vi "Function 1.vi"(8 "error in (no error)":errorcluster, 10 "Differential_Top":dbl=10.0 format="%#_13g", 11 "Data Cluster":T1={"Vesta Data Output"={"Temp_W_Raw_U"=0, "Temp_W_Raw_L"=0, "Temperature Water (F)"=0.0, "Temperature Water Compensated (F)"=0.0, "Temperature Ambient (F)"=0.0, "Setpoint Location (F)"=0.0, "Heat Request"="", "Fault Ram"="", "PWM DCDC Value"=0, "Pilot Voltage (mV)"=0.0, "Setpoint Actual (F)"=0.0, "Differential Actual (F)"=0.0, "Setpoint User (F)"=0.0, "Differential User (F)"=0.0, "Termperature FIltered -TCO (F)"=0.0, "Temp_C_Raw_1 - Sensor Voltage"="", "Temp_C_Raw_2 - Sensor Voltage"="", "Chamber Sensor Temperature (F)"=0.0, "LDO Base Temperature (F)"=0.0, "LDO Timer (sec)"=0, "Disabled (0)"=FALSE, "Warming (1)"=FALSE, "Heating (2)"=FALSE, "Cooling Data Write (3)"=FALSE, "Cooling (4)"=FALSE, "Data Read (5)"=FALSE, "N/A"=FALSE, "Temperature Trip (7)"=FALSE, "Burner"=FALSE}, "VestaTemperature"={"Water Heater Temp (°F)"=135, "Differential  (°F)"=10.0}, "Timer Application Data"={"Duty Cycle"={"Burner ON Time (Seconds)"=60.0, "Burner OFF Time (Seconds)"=60.0, "Main Burner Flag"=FALSE, "Burner Power Mode"=0}}, "Data Array"=[], "MW Output"={"TC1-Channel 021"=0.0, "TC2-Channel 022"=0.0, "TC3-Channel 023"=0.0, "TC4-Channel 024"=0.0, "TC5-Channel 025"=0.0, "TC6-Channel 026"=0.0, "TC7-Channel 017"=0.0, "TC8-Channel 028"=0.0, "TC9-Channel 029"=0.0, "TC10-Channel 030"=0.0, "TC Tree Average"=0.0, "TC DWN- Channel 027"=0.0, "RTDin-Channel 031"=0.0, "RTDout-Channel 032"=0.0, "RTDamb-Channel 033"=0.0, "PSI1-Channel 011"=0.0, "PSI2-Channel 012"=0.0, "PSI3-Channel 013"=0.0, "PSI4-Channel 014"=0.0, "UE State-Channel 015"=0.0, "LE State-Channel 016"=0.0, "Module 4 Relay Status Output"={"INTELLIFAUCET TEMP(T)/FLOW(F) (CH 041)"=FALSE, "INTELLIFAUCET READY (CH 042)"=FALSE, "INTELLIFAUCET START (CH 043)"=FALSE, "INTELLIFAUCET STOP (CH 044)"=FALSE, "MAIN POWER RELAY (CH 047)"=FALSE, "NOT USED (CH 045)"=FALSE, "NOT USED (CH 046)"=FALSE, "PURGE VALVE RELAY (CH 048)"=FALSE, "OUTLET VALVE RELAY (CH 049)"=FALSE, "INLET VALVE RELAY (CH 050)"=FALSE, "Intellifaucet (% Open)"=0.0, "Proportioning Valve (%Open)"=0.0, "Intellifaucet Temp Setpoint (F)"=0.0}}} {"VestaTemperature"."Water Heater Temp (°F)" min=32 max=203}) -> (0 "error out":errorcluster, 3 "Data Cluster Out":T1={"Vesta Data Output"={"Temp_W_Raw_U"=0, "Temp_W_Raw_L"=0, "Temperature Water (F)"=0.0, "Temperature Water Compensated (F)"=0.0, "Temperature Ambient (F)"=0.0, "Setpoint Location (F)"=0.0, "Heat Request"="", "Fault Ram"="", "PWM DCDC Value"=0, "Pilot Voltage (mV)"=0.0, "Setpoint Actual (F)"=0.0, "Differential Actual (F)"=0.0, "Setpoint User (F)"=0.0, "Differential User (F)"=0.0, "Termperature FIltered -TCO (F)"=0.0, "Temp_C_Raw_1 - Sensor Voltage"="", "Temp_C_Raw_2 - Sensor Voltage"="", "Chamber Sensor Temperature (F)"=0.0, "LDO Base Temperature (F)"=0.0, "LDO Timer (sec)"=0, "Disabled (0)"=FALSE, "Warming (1)"=FALSE, "Heating (2)"=FALSE, "Cooling Data Write (3)"=FALSE, "Cooling (4)"=FALSE, "Data Read (5)"=FALSE, "N/A"=FALSE, "Temperature Trip (7)"=FALSE, "Burner"=FALSE}, "VestaTemperature"={"Water Heater Temp (°F)"=135, "Differential  (°F)"=10.0}, "Timer Application Data"={"Duty Cycle"={"Burner ON Time (Seconds)"=60.0, "Burner OFF Time (Seconds)"=60.0, "Main Burner Flag"=FALSE, "Burner Power Mode"=0}}, "Data Array"=[], "MW Output"={"TC1-Channel 021"=0.0, "TC2-Channel 022"=0.0, "TC3-Channel 023"=0.0, "TC4-Channel 024"=0.0, "TC5-Channel 025"=0.0, "TC6-Channel 026"=0.0, "TC7-Channel 017"=0.0, "TC8-Channel 028"=0.0, "TC9-Channel 029"=0.0, "TC10-Channel 030"=0.0, "TC Tree Average"=0.0, "TC DWN- Channel 027"=0.0, "RTDin-Channel 031"=0.0, "RTDout-Channel 032"=0.0, "RTDamb-Channel 033"=0.0, "PSI1-Channel 011"=0.0, "PSI2-Channel 012"=0.0, "PSI3-Channel 013"=0.0, "PSI4-Channel 014"=0.0, "UE State-Channel 015"=0.0, "LE State-Channel 016"=0.0, "Module 4 Relay Status Output"={"INTELLIFAUCET TEMP(T)/FLOW(F) (CH 041)"=FALSE, "INTELLIFAUCET READY (CH 042)"=FALSE, "INTELLIFAUCET START (CH 043)"=FALSE, "INTELLIFAUCET STOP (CH 044)"=FALSE, "MAIN POWER RELAY (CH 047)"=FALSE, "NOT USED (CH 045)"=FALSE, "NOT USED (CH 046)"=FALSE, "PURGE VALVE RELAY (CH 048)"=FALSE, "OUTLET VALVE RELAY (CH 049)"=FALSE, "INLET VALVE RELAY (CH 050)"=FALSE, "Intellifaucet (% Open)"=0.0, "Proportioning Valve (%Open)"=0.0, "Intellifaucet Temp Setpoint (F)"=0.0}}} {"VestaTemperature"."Water Heater Temp (°F)" min=32 max=203}, 4 "Send_Vesta_Message":u8)   [LabVIEW 2023]
uses:
  controls/UI Data.ctl
  Drivers/Resideo Gas Valve/Type Definitions/Vesta Info.ctl
  Drivers/Resideo Gas Valve/Type Definitions/Temperature Control.ctl
  controls/Timer Application Cluster.ctl
  controls/Burner Duty Cycle.ctl
  Hybrid Water Heater/Type Definitions/HEWH MW100 Data Cluster.ctl
  Hybrid Water Heater/Custom Instrument Control/MW100/Type Definitions/HEWH Module 4 Relay Status.ctl
  <vilib>/Utility/error.llb/whitespace.ctl
  <vilib>/Utility/error.llb/Trim Whitespace One-Sided.vi
panel:
  out "Burner":i16
  out "Power_Mode_Out":u8
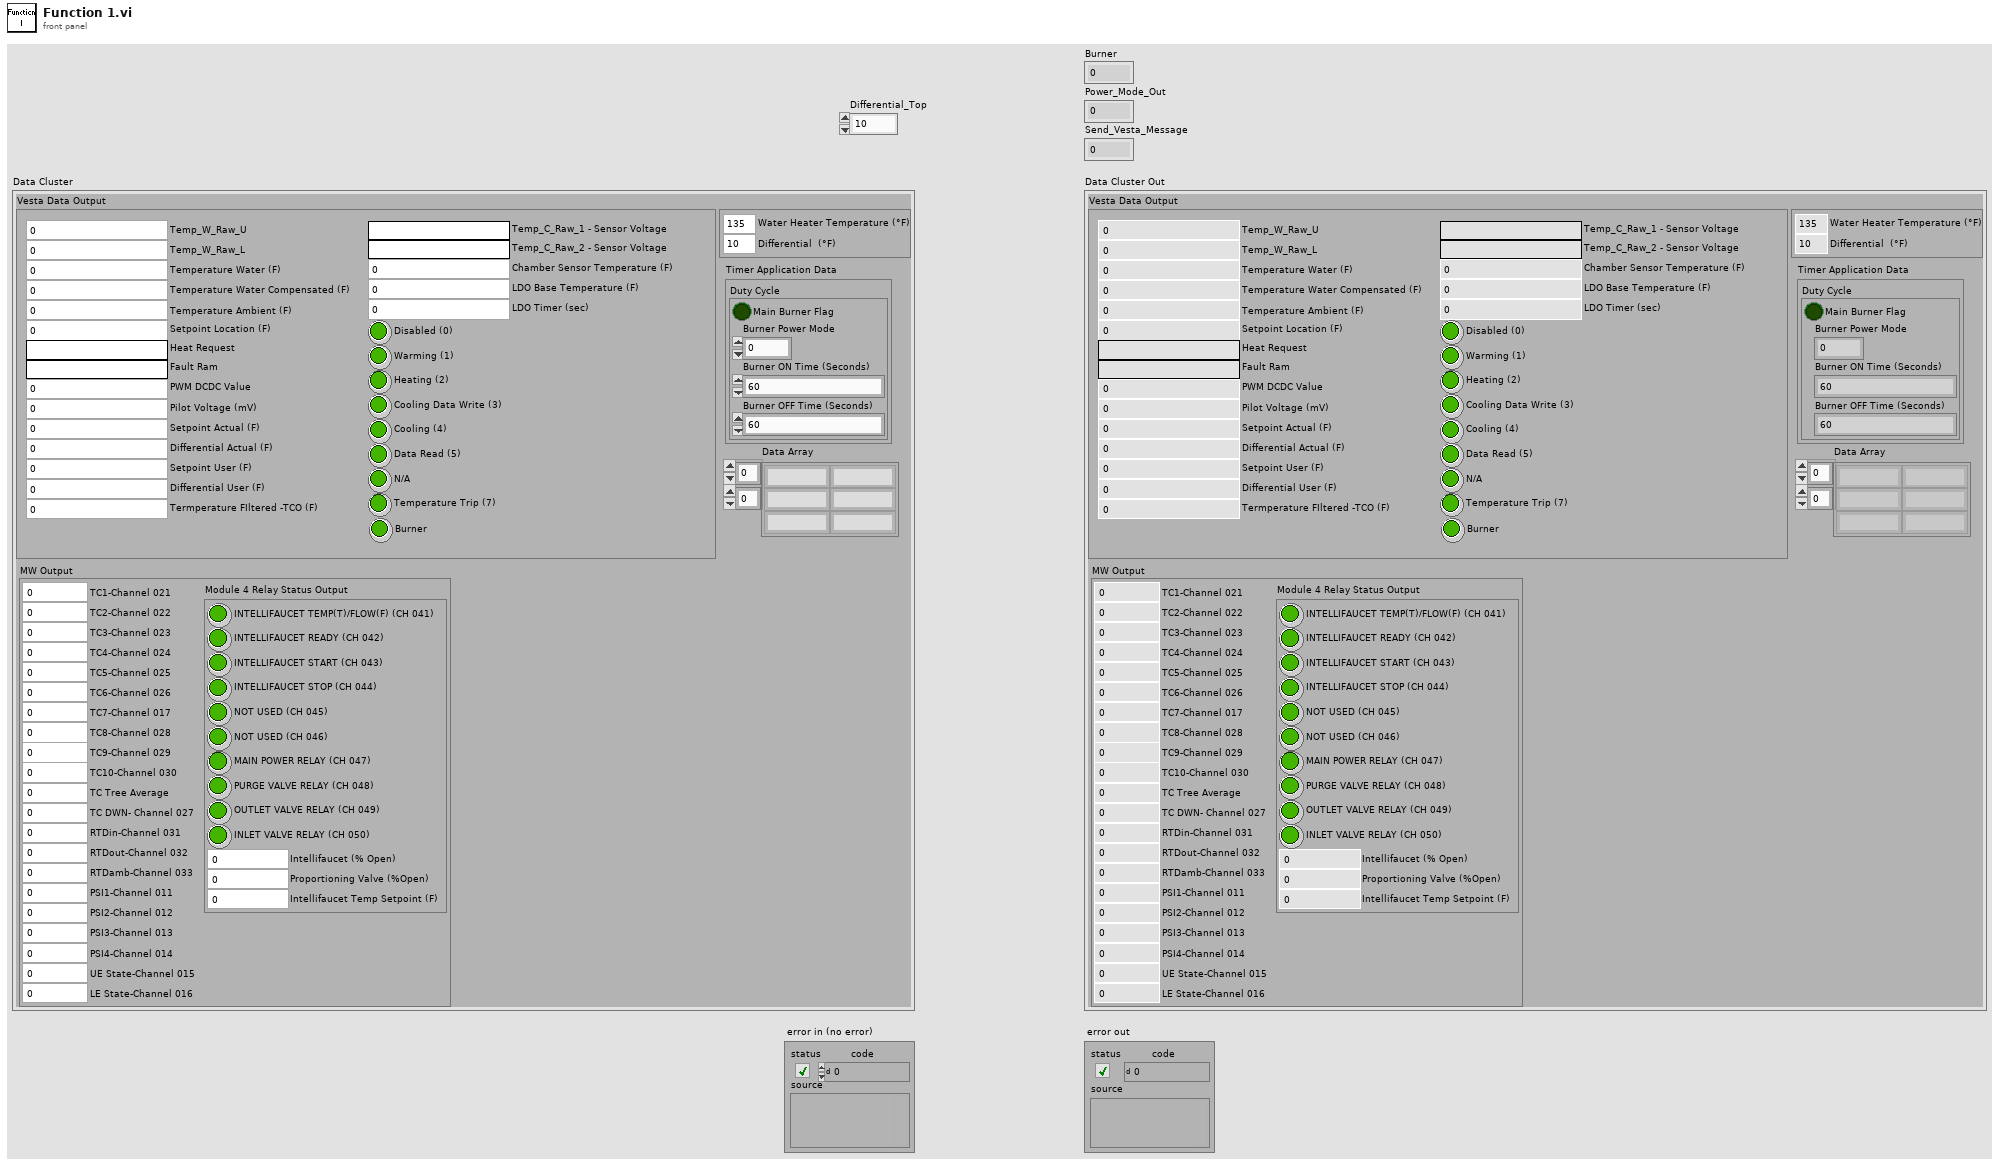
[diagram p1: front panel]
types:
  T1 = typedef "UI Data.ctl" = cluster{"Vesta Data Output":T2, "VestaTemperature":T3, "Timer Application Data":T4, "Data Array":string[][], "MW Output":T6}
  T2 = typedef "Vesta Info.ctl" = cluster{"Temp_W_Raw_U":u16, "Temp_W_Raw_L":u16, "Temperature Water (F)":dbl, "Temperature Water Compensated (F)":dbl, "Temperature Ambient (F)":dbl, "Setpoint Location (F)":dbl, "Heat Request":string, "Fault Ram":string, "PWM DCDC Value":u16, "Pilot Voltage (mV)":dbl, "Setpoint Actual (F)":dbl, "Differential Actual (F)":dbl, "Setpoint User (F)":dbl, "Differential User (F)":dbl, "Termperature FIltered -TCO (F)":dbl, "Temp_C_Raw_1 - Sensor Voltage":string, "Temp_C_Raw_2 - Sensor Voltage":string, "Chamber Sensor Temperature (F)":dbl, "LDO Base Temperature (F)":dbl, "LDO Timer (sec)":i16, "Disabled (0)":bool, "Warming (1)":bool, "Heating (2)":bool, "Cooling Data Write (3)":bool, "Cooling (4)":bool, "Data Read (5)":bool, "N/A":bool, "Temperature Trip (7)":bool, "Burner":bool}
  T3 = typedef "Temperature Control.ctl" = cluster{"Water Heater Temp (°F)":u16, "Differential  (°F)":dbl}
  T4 = typedef "Timer Application Cluster.ctl" = cluster{"Duty Cycle":T5}
  T5 = typedef "Burner Duty Cycle.ctl" = cluster{"Burner ON Time (Seconds)":dbl, "Burner OFF Time (Seconds)":dbl, "Main Burner Flag":bool, "Burner Power Mode":u8}
  T6 = typedef "HEWH MW100 Data Cluster.ctl" = cluster{"TC1-Channel 021":dbl, "TC2-Channel 022":dbl, "TC3-Channel 023":dbl, "TC4-Channel 024":dbl, "TC5-Channel 025":dbl, "TC6-Channel 026":dbl, "TC7-Channel 017":dbl, "TC8-Channel 028":dbl, "TC9-Channel 029":dbl, "TC10-Channel 030":dbl, "TC Tree Average":dbl, "TC DWN- Channel 027":dbl, "RTDin-Channel 031":dbl, "RTDout-Channel 032":dbl, "RTDamb-Channel 033":dbl, "PSI1-Channel 011":dbl, "PSI2-Channel 012":dbl, "PSI3-Channel 013":dbl, "PSI4-Channel 014":dbl, "UE State-Channel 015":dbl, "LE State-Channel 016":dbl, "Module 4 Relay Status Output":T7}
  T7 = typedef "HEWH Module 4 Relay Status.ctl" = cluster{"INTELLIFAUCET TEMP(T)/FLOW(F) (CH 041)":bool, "INTELLIFAUCET READY (CH 042)":bool, "INTELLIFAUCET START (CH 043)":bool, "INTELLIFAUCET STOP (CH 044)":bool, "MAIN POWER RELAY (CH 047)":bool, "NOT USED (CH 045)":bool, "NOT USED (CH 046)":bool, "PURGE VALVE RELAY (CH 048)":bool, "OUTLET VALVE RELAY (CH 049)":bool, "INLET VALVE RELAY (CH 050)":bool, "Intellifaucet (% Open)":dbl, "Proportioning Valve (%Open)":dbl, "Intellifaucet Temp Setpoint (F)":dbl}
  T8 = typedef "whitespace.ctl" = u16
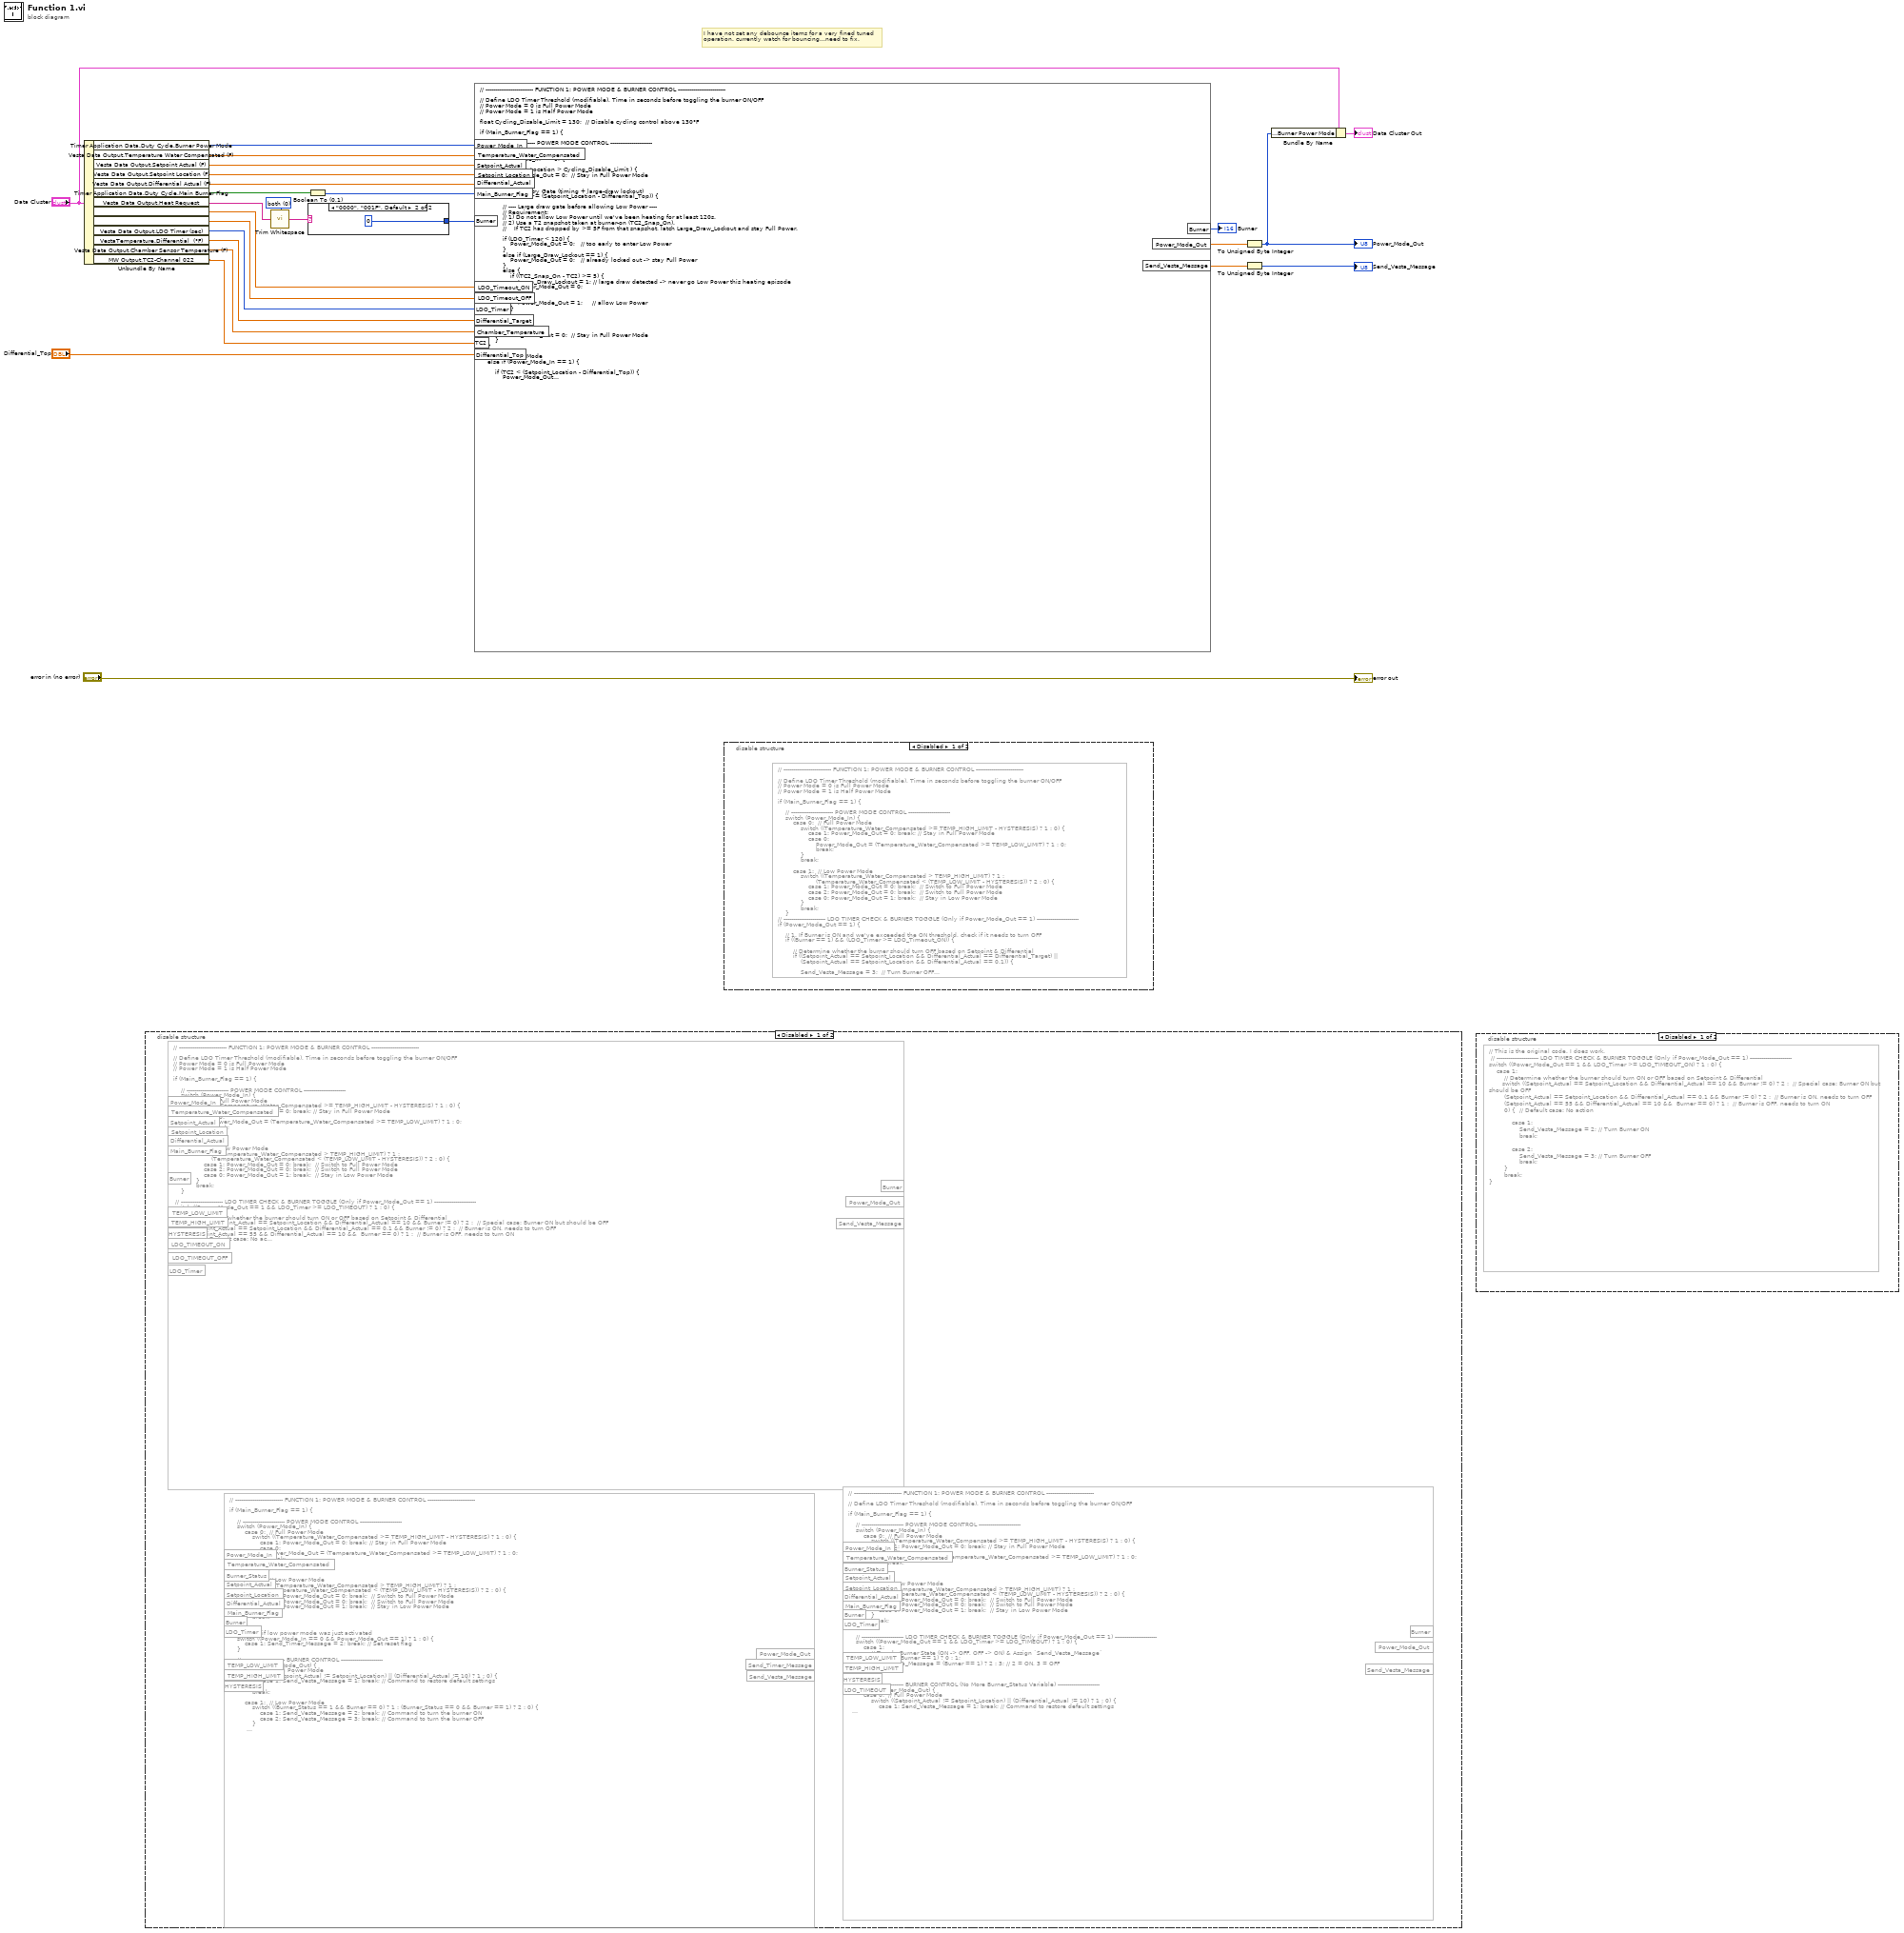
[diagram p0: block diagram]
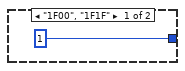
[diagram p4: hidden frame]
diagram:
  w9 = T8 0 items=["both", "start of string", "end of string"] ("location (both)")
  # "I have not set any debounce items for a very fined tuned \noperation. currently watch for bouncing...need to fix."
  n1 = Unbundle By Name("Data Cluster") -> ("Timer Application Data.Duty Cycle.Burner Power Mode"=w20:u8, "Vesta Data Output.Temperature Water Compensated (F)"=w19:dbl, "Vesta Data Output.Setpoint Actual (F)"=w24:dbl, "Vesta Data Output.Setpoint Location (F)"=w23:dbl, "Vesta Data Output.Differential Actual (F)"=w22:dbl, "Timer Application Data.Duty Cycle.Main Burner Flag"=w26:bool, "Vesta Data Output.Heat Request"=w10:string, "Timer Application Data.Duty Cycle.Burner ON Time (Seconds)"=w7:dbl, "Timer Application Data.Duty Cycle.Burner OFF Time (Seconds)"=w6:dbl, "Vesta Data Output.LDO Timer (sec)"=w12:i16, "VestaTemperature.Differential  (°F)"=w4:dbl, "Vesta Data Output.Chamber Sensor Temperature (F)"=w3:dbl, "MW Output.TC2-Channel 022"=w2:dbl)
  n2 = disable-structure shown="Disabled" {
    frame Disabled {
      n3 = formula code="// ------------------------- FUNCTION 1: POWER MODE & BURNER CONTROL -------------------------\n\n// Define LDO Timer Threshold (modifiable), Time in seconds before toggling the burner ON/OFF\n// Power Mode = 0 is Full Power Mode\n// Power Mode = 1 is Half Power Mode\n\nif (Main_Burner_Flag == 1) {\n\n    // ---------------------- POWER MODE CONTROL ----------------------\n    switch (Power_Mode_In) {\n        case 0:  // Full Power Mode\n            switch ((Temperature_Water_Compensated >= TEMP_HIGH_LIMIT - HYSTERESIS) ? 1 : 0) {\n                case 1: Power_Mode_Out = 0; break; // Stay in Full Power Mode\n                case 0:\n                    Power_Mode_Out = (Temperature_Water_Compensated >= TEMP_LOW_LIMIT) ? 1 : 0;\n                    break;\n            }\n            break;\n\n        case 1:  // Low Power Mode\n            switch ((Temperature_Water_Compensated > TEMP_HIGH_LIMIT) ? 1 : \n                    (Temperature_Water_Compensated < (TEMP_LOW_LIMIT - HYSTERESIS)) ? 2 : 0) {\n                case 1: Power_Mode_Out = 0; break;  // Switch to Full Power Mode\n                case 2: Power_Mode_Out = 0; break;  // Switch to Full Power Mode\n                case 0: Power_Mode_Out = 1; break;  // Stay in Low Power Mode\n            }\n            break;\n    }\n\n // ---------------------- LDO TIMER CHECK & BURNER TOGGLE (Only if Power_Mode_Out == 1) ----------------------\nswitch ((Power_Mode_Out == 1 && LDO_Timer >= LDO_TIMEOUT) ? 1 : 0) {\n    case 1:\n        // Determine whether the burner should turn ON or OFF based on Setpoint & Differential\n       switch ((Setpoint_Actual == Setpoint_Location && Differential_Actual == 10 && Burner != 0) ? 2 :  // Special case: Burner ON but should be OFF\n        (Setpoint_Actual == Setpoint_Location && Differential_Actual == 0.1 && Burner != 0) ? 2 :  // Burner is ON, needs to turn OFF\n        (Setpoint_Actual == 55 && Differential_Actual == 10 &&  Burner == 0) ? 1 :  // Burner is OFF, needs to turn ON\n        0) {  // Default case: No action\n\n            case 1:  \n                Send_Vesta_Message = 2; // Turn Burner ON\n                break;\n\n            case 2:\n                Send_Vesta_Message = 3; // Turn Burner OFF\n                break;\n        }\n        break;\n}\n\n    // ---------------------- BURNER CONTROL (No More Burner_Status Variable) ----------------------\n    switch (Power_Mode_Out) {\n        case 0:  // Full Power Mode\n            switch ((Setpoint_Actual != Setpoint_Location) || (Differential_Actual != 10) ? 1 : 0) {\n                case 1: Send_Vesta_Message = 1; break; // Command to restore default settings\n            }\n            break;\n    }\n}"() -> ()  [unwired: 13 in, 3 out]
      n4 = formula code="// ------------------------- FUNCTION 1: POWER MODE & BURNER CONTROL -------------------------\n\nif (Main_Burner_Flag == 1) {\n\n    // ---------------------- POWER MODE CONTROL ----------------------\n    switch (Power_Mode_In) {\n        case 0:  // Full Power Mode\n            switch ((Temperature_Water_Compensated >= TEMP_HIGH_LIMIT - HYSTERESIS) ? 1 : 0) {\n                case 1: Power_Mode_Out = 0; break; // Stay in Full Power Mode\n                case 0:\n                    Power_Mode_Out = (Temperature_Water_Compensated >= TEMP_LOW_LIMIT) ? 1 : 0;\n                    break;\n            }\n            break;\n\n        case 1:  // Low Power Mode\n            switch ((Temperature_Water_Compensated > TEMP_HIGH_LIMIT) ? 1 : \n                    (Temperature_Water_Compensated < (TEMP_LOW_LIMIT - HYSTERESIS)) ? 2 : 0) {\n                case 1: Power_Mode_Out = 0; break;  // Switch to Full Power Mode\n                case 2: Power_Mode_Out = 0; break;  // Switch to Full Power Mode\n                case 0: Power_Mode_Out = 1; break;  // Stay in Low Power Mode\n            }\n            break;\n    }\n\n    // Check if low power mode was just activated\n    switch ((Power_Mode_In == 0 && Power_Mode_Out == 1) ? 1 : 0) {\n        case 1: Send_Timer_Message = 2; break; // Set reset flag\n    }\n\n    // ---------------------- BURNER CONTROL ----------------------\n    switch (Power_Mode_Out) {\n        case 0:  // Full Power Mode\n            switch ((Setpoint_Actual != Setpoint_Location) || (Differential_Actual != 10) ? 1 : 0) {\n                case 1: Send_Vesta_Message = 1; break; // Command to restore default settings\n            }\n            break;\n\n        case 1:  // Low Power Mode\n            switch ((Burner_Status == 1 && Burner == 0) ? 1 : (Burner_Status == 0 && Burner == 1) ? 2 : 0) {\n                case 1: Send_Vesta_Message = 2; break; // Command to turn the burner ON\n                case 2: Send_Vesta_Message = 3; break; // Command to turn the burner OFF\n            }\n            break;\n    }\n}"() -> ()  [unwired: 12 in, 3 out]
      n5 = formula code="// ------------------------- FUNCTION 1: POWER MODE & BURNER CONTROL -------------------------\n\n// Define LDO Timer Threshold (modifiable), Time in seconds before toggling the burner ON/OFF\n\nif (Main_Burner_Flag == 1) {\n\n    // ---------------------- POWER MODE CONTROL ----------------------\n    switch (Power_Mode_In) {\n        case 0:  // Full Power Mode\n            switch ((Temperature_Water_Compensated >= TEMP_HIGH_LIMIT - HYSTERESIS) ? 1 : 0) {\n                case 1: Power_Mode_Out = 0; break; // Stay in Full Power Mode\n                case 0:\n                    Power_Mode_Out = (Temperature_Water_Compensated >= TEMP_LOW_LIMIT) ? 1 : 0;\n                    break;\n            }\n            break;\n\n        case 1:  // Low Power Mode\n            switch ((Temperature_Water_Compensated > TEMP_HIGH_LIMIT) ? 1 : \n                    (Temperature_Water_Compensated < (TEMP_LOW_LIMIT - HYSTERESIS)) ? 2 : 0) {\n                case 1: Power_Mode_Out = 0; break;  // Switch to Full Power Mode\n                case 2: Power_Mode_Out = 0; break;  // Switch to Full Power Mode\n                case 0: Power_Mode_Out = 1; break;  // Stay in Low Power Mode\n            }\n            break;\n    }\n\n    // ---------------------- LDO TIMER CHECK & BURNER TOGGLE (Only if Power_Mode_Out == 1) ----------------------\n    switch ((Power_Mode_Out == 1 && LDO_Timer >= LDO_TIMEOUT) ? 1 : 0) {\n        case 1:\n            // Toggle Burner State (ON -> OFF, OFF -> ON) & Assign `Send_Vesta_Message`\n            Burner = (Burner == 1) ? 0 : 1;\n            Send_Vesta_Message = (Burner == 1) ? 2 : 3; // 2 = ON, 3 = OFF\n            break;\n    }\n\n    // ---------------------- BURNER CONTROL (No More Burner_Status Variable) ----------------------\n    switch (Power_Mode_Out) {\n        case 0:  // Full Power Mode\n            switch ((Setpoint_Actual != Setpoint_Location) || (Differential_Actual != 10) ? 1 : 0) {\n                case 1: Send_Vesta_Message = 1; break; // Command to restore default settings\n            }\n            break;\n    }\n}"() -> ()  [unwired: 13 in, 3 out]
    }
    frame Enabled {
    }
  }
  n6 = call <vilib>:"Trim Whitespace.vi"("string"=w10, "location (both)"=w9) -> ("trimmed string"=w8:string)
  n7 = case shown="\"0000\", \"001F\", Default" w8 {
    tunnel: [1 0] -> w11
    frame "1F00", "1F1F" {
    }
    frame "0000", "001F", Default {
    }
  }
  n8 = Boolean To (0,1)(Boolean=w26) -> (0, 1=w21:i16)
  n9 = formula code="// ------------------------- FUNCTION 1: POWER MODE & BURNER CONTROL -------------------------\n\n// Define LDO Timer Threshold (modifiable), Time in seconds before toggling the burner ON/OFF\n// Power Mode = 0 is Full Power Mode\n// Power Mode = 1 is Half Power Mode\n\nfloat Cycling_Disable_Limit = 130;  // Disable cycling control above 130°F\n\nif (Main_Burner_Flag == 1) {\n\n    // ---------------------- POWER MODE CONTROL ----------------------\n    \n   // Full Power Mode\n    if (Power_Mode_In == 0) {  \n        \n        if (Setpoint_Location > Cycling_Disable_Limit ) {\n            Power_Mode_Out = 0;  // Stay in Full Power Mode\n        }  \n\n   // Low Power Entry Gate (timing + large-draw lockout)\n        else if (TC2 >= (Setpoint_Location - Differential_Top)) {\n\n            // ---- Large draw gate before allowing Low Power ----\n            // Requirement:\n            // 1) Do not allow Low Power until we've been heating for at least 120s.\n            // 2) Use a T2 snapshot taken at burner-on (TC2_Snap_On).\n            //    If TC2 has dropped by >= 5F from that snapshot, latch Large_Draw_Lockout and stay Full Power.\n\n            if (LDO_Timer < 120) {\n                Power_Mode_Out = 0;   // too early to enter Low Power\n            }\n            else if (Large_Draw_Lockout == 1) {\n                Power_Mode_Out = 0;   // already locked out -> stay Full Power\n            }\n            else {\n                if ((TC2_Snap_On - TC2) >= 5) {\n                    Large_Draw_Lockout = 1; // large draw detected -> never go Low Power this heating episode\n                    Power_Mode_Out = 0;\n                } \n                else {\n                    Power_Mode_Out = 1;     // allow Low Power\n                }\n            }\n        }\n       \n        else {\n            Power_Mode_Out = 0;  // Stay in Full Power Mode\n        }\n    } \n\n    // Low Power Mode\n    else if (Power_Mode_In == 1) { \n \n        if (TC2 < (Setpoint_Location - Differential_Top)) {\n            Power_Mode_Out = 0;  // Too cold at top -> go back to Full Power (recovery)\n        } \n        else if (TC2 >= Setpoint_Location) {\n            Power_Mode_Out = 0;  // Setpoint reached, exit Low Power Mode\n        }\n        else {\n            Power_Mode_Out = 1;  // Stay in Low Power Mode\n        }\n    }\n}\nelse {Power_Mode_Out = 0;}   // If Main_Burner_Flag ==0, then Power_Mode_Out ==0;\n\n// ---------------------- LDO TIMER CHECK & BURNER TOGGLE (Only if Power_Mode_Out == 1) ----------------------\n// Burner duty cycling corresponds to a generalized combustion-chamber temperature.\n// Right now it’s controlled by a basic timer, but it can be tuned to target a specific temperature.\n// Potentially this could use a table lookup to maximize thermal heat transfer.\n\nif (Power_Mode_Out == 1) {\n\n    // 1. If Burner is ON and we've exceeded the ON threshold, check if it needs to turn OFF\n    if ((Burner == 1) && (LDO_Timer >= LDO_Timeout_ON)) {\n\n        // Determine whether the burner should turn OFF based on Setpoint & Differential\n        if ((Setpoint_Actual == Setpoint_Location && Differential_Actual == Differential_Target) ||\n            (Setpoint_Actual == Setpoint_Location && Differential_Actual == 0.1)) {\n\n            Send_Vesta_Message = 3;  // Turn Burner OFF\n        }\n    }\n\n    // 2. Else if Burner is OFF and we've exceeded the OFF threshold, check if it needs to turn ON\n    else if ((Burner == 0) && (LDO_Timer >= LDO_Timeout_OFF)) {\n\n        // Determine whether the burner should turn ON based on Setpoint & Differential\n        if ((Setpoint_Actual == 55) && (Differential_Actual == Differential_Target)) {\n\n            Send_Vesta_Message = 2;  // Turn Burner ON\n        }\n    }\n}\n\n// ---------------------- BURNER CONTROL (No More Burner_Status Variable) ----------------------\nif (Power_Mode_Out == 0) {  // Full Power Mode\n    \n    if ((Setpoint_Actual != Setpoint_Location) || (Differential_Actual != Differential_Target)) {\n        Send_Vesta_Message = 1;  // Command to restore default settings\n    }\n}"("Power_Mode_In"=w20, "Temperature_Water_Compensated"=w19, "Main_Burner_Flag"=w21, "Setpoint_Actual"=w24, "Setpoint_Location"=w23, "Differential_Actual"=w22, "Burner"=w11, "LDO_Timer"=w12, "LDO_Timeout_ON"=w7, "LDO_Timeout_OFF"=w6, "Differential_Target"=w4, "Chamber_Temperature"=w3, "TC2"=w2, "Differential_Top"="Differential_Top") -> ("Power_Mode_Out"=w16:dbl, "Send_Vesta_Message"=w18:dbl, "Burner"=→"Burner":i32)
  n10 = disable-structure shown="Disabled" {
    frame Disabled {
      n11 = formula code="// ------------------------- FUNCTION 1: POWER MODE & BURNER CONTROL -------------------------\n\n// Define LDO Timer Threshold (modifiable), Time in seconds before toggling the burner ON/OFF\n// Power Mode = 0 is Full Power Mode\n// Power Mode = 1 is Half Power Mode\n\nif (Main_Burner_Flag == 1) {\n\n    // ---------------------- POWER MODE CONTROL ----------------------\n    switch (Power_Mode_In) {\n        case 0:  // Full Power Mode\n            switch ((Temperature_Water_Compensated >= TEMP_HIGH_LIMIT - HYSTERESIS) ? 1 : 0) {\n                case 1: Power_Mode_Out = 0; break; // Stay in Full Power Mode\n                case 0:\n                    Power_Mode_Out = (Temperature_Water_Compensated >= TEMP_LOW_LIMIT) ? 1 : 0;\n                    break;\n            }\n            break;\n\n        case 1:  // Low Power Mode\n            switch ((Temperature_Water_Compensated > TEMP_HIGH_LIMIT) ? 1 : \n                    (Temperature_Water_Compensated < (TEMP_LOW_LIMIT - HYSTERESIS)) ? 2 : 0) {\n                case 1: Power_Mode_Out = 0; break;  // Switch to Full Power Mode\n                case 2: Power_Mode_Out = 0; break;  // Switch to Full Power Mode\n                case 0: Power_Mode_Out = 1; break;  // Stay in Low Power Mode\n            }\n            break;\n    }\n// ---------------------- LDO TIMER CHECK & BURNER TOGGLE (Only if Power_Mode_Out == 1) ----------------------\nif (Power_Mode_Out == 1) {\n\n    // 1. If Burner is ON and we've exceeded the ON threshold, check if it needs to turn OFF\n    if ((Burner == 1) && (LDO_Timer >= LDO_Timeout_ON)) {\n\n        // Determine whether the burner should turn OFF based on Setpoint & Differential\n        if ((Setpoint_Actual == Setpoint_Location && Differential_Actual == Differential_Target) ||\n            (Setpoint_Actual == Setpoint_Location && Differential_Actual == 0.1)) {\n\n            Send_Vesta_Message = 3;  // Turn Burner OFF\n        }\n    }\n\n    // 2. Else if Burner is OFF and we've exceeded the OFF threshold, check if it needs to turn ON\n    else if ((Burner == 0) && (LDO_Timer >= LDO_Timeout_OFF)) {\n\n        // Determine whether the burner should turn ON based on Setpoint & Differential\n        if ((Setpoint_Actual == 55) && (Differential_Actual == Differential_Target)) {\n\n            Send_Vesta_Message = 2;  // Turn Burner ON\n        }\n    }\n}\n    // ---------------------- BURNER CONTROL (No More Burner_Status Variable) ----------------------\n    switch (Power_Mode_Out) {\n        case 0:  // Full Power Mode\n            switch ((Setpoint_Actual != Setpoint_Location) || (Differential_Actual != Differential_Target) ? 1 : 0) {\n                case 1: Send_Vesta_Message = 1; break; // Command to restore default settings\n            }\n            break;\n    }\n}"() -> ()
    }
    frame Enabled {
    }
  }
  n12 = To Unsigned Byte Integer(number=w16) -> (unsigned 8bit integer=w13:u8)
  "Power_Mode_Out" <- w13
  n13 = To Unsigned Byte Integer(number=w18) -> (unsigned 8bit integer=→"Send_Vesta_Message":u8)
  n14 = Bundle By Name(cluster="Data Cluster", "Timer Application Data.Duty Cycle.Burner Power Mode"=w13) -> (→"Data Cluster Out":T1)
  n15 = disable-structure shown="Disabled" {
    frame Disabled {
      n16 = formula code="// This is the original code. I does work. \n // ---------------------- LDO TIMER CHECK & BURNER TOGGLE (Only if Power_Mode_Out == 1) ----------------------\nswitch ((Power_Mode_Out == 1 && LDO_Timer >= LDO_TIMEOUT_ON) ? 1 : 0) {\n    case 1:\n        // Determine whether the burner should turn ON or OFF based on Setpoint & Differential\n       switch ((Setpoint_Actual == Setpoint_Location && Differential_Actual == 10 && Burner != 0) ? 2 :  // Special case: Burner ON but should be OFF\n        (Setpoint_Actual == Setpoint_Location && Differential_Actual == 0.1 && Burner != 0) ? 2 :  // Burner is ON, needs to turn OFF\n        (Setpoint_Actual == 55 && Differential_Actual == 10 &&  Burner == 0) ? 1 :  // Burner is OFF, needs to turn ON\n        0) {  // Default case: No action\n\n            case 1:  \n                Send_Vesta_Message = 2; // Turn Burner ON\n                break;\n\n            case 2:\n                Send_Vesta_Message = 3; // Turn Burner OFF\n                break;\n        }\n        break;\n}"() -> ()
    }
    frame Enabled {
    }
  }
  "error out" <- "error in (no error)"
